vi "MonoSpec50 WavelgtDialog.vi"(4 "error in (no error)":errorcluster, 6 "PosAct":dbl caption="Position \nActuelle (nm)") -> (0 "error out":errorcluster, 2 "PosAct Out":dbl caption="Position \nActuelle (nm)")   [LabVIEW 2012]
doc: "Ce VI permet la saisie de la position actuelle, en nm, telle qu'indiquée sur l'affichage à roulette du Monospec 50"
panel:
  in  "OK Button":bool
  # "Entrez la position actuelle du monochromateur,\ntel qu'indiquée sur l'affichage à roulette"
  # "**La position indiqué sur l'affichage à roulette du MonoSpec 50 est spécifié en Armstrong(Å). Veillez à diviser cette position par 10. \nEx.: Affichage : 5001 -> position à entrer : 500,1 nm"
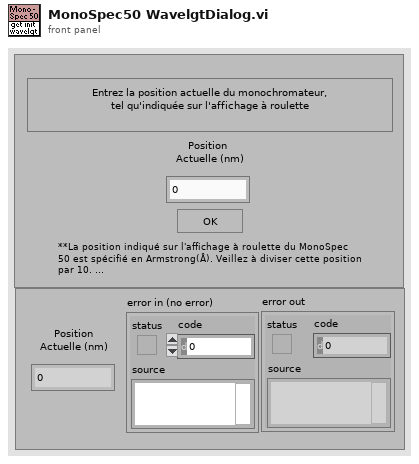
[diagram p1: front panel]
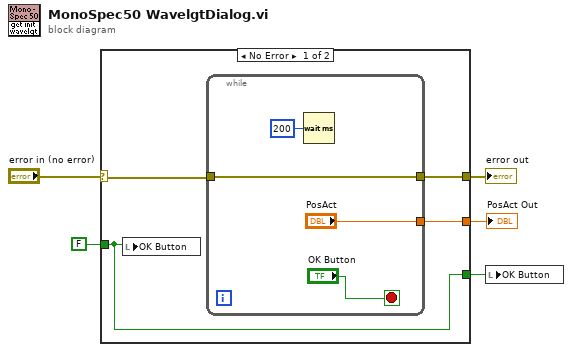
[diagram p0: block diagram]
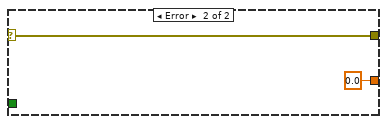
[diagram p2: hidden frame]
diagram:
  n1 = case shown="No Error" "error in (no error)" {
    selector: "error in (no error)" -> [w7 w15]
    tunnel: [w8 w15] -> w4
    tunnel: [w9 0.0 ("PosAct")] -> w3
    tunnel: FALSE ("OK Button") -> [w6 _]
    tunnel: [w6 _] -> w1
    frame No Error {
      n2 = local write "OK Button"(w6) -> ()
      n3 = while {
        tunnel: w7 -> [w11]
        tunnel: [w11] -> w8
        tunnel: ["PosAct"] -> w9
        stop <- "OK Button" stop-if-true
        n4 = Wait (ms)(milliseconds to wait=u32 200) -> ()  [unwired: 1 out]
      }
    }
    frame Error {
    }
  }
  "error out" <- w4
  "PosAct Out" <- w3
  n5 = local write "OK Button"(w1) -> ()
